vi "KE6514.constructor.vi"(0 "name":string, 2 "data in":string, 5 "error in (no error)":errorcluster) -> (14 "i ref out":refnum<vi>, 16 "data out":string, 19 "error out":errorcluster)   [LabVIEW 2014, in "KE6514.lvlib"]
doc: "This is the constructor of a class.\n\nLicense Agreement for this software:\n\nCopyright (C)\nGesellschaft für Schwerionenforschung, GSI\nPlanckstr. 1\n64291 Darmstadt\nGermany\n\nContact: D.Beck@gsi.de \n\nThis program is free software; you can redistribute it and/or modify it under the terms of the \nGNU General Public License as published by the Free Software Foundation; either version 2 of \nthe license, or (at your option) any later version.\n\nThis program is distributed in the hope that it will be useful, but WITHOUT ANY WARRANTY; \nwithout even the implied warranty of MERCHANTABILITY or FITNESS FOR A PARTICULAR PURPOSE. See the GNU General License for more details (http://www.gnu.org).\n\nGesellschaft für Schwerionenforschung, GSI\nPlanckstr. 1, 64291 Darmstadt, Germany\nFor all questions and ideas contact: M.Richter@gsi.de, H.Brand@gsi.de or D.Beck@gsi.de.\nLast update: 16-JUN-2004"
uses:
  KE6514.lvlib
  CSCore/CSApplicationBaseClasses/DeviceBase/DeviceBase.myEventNames.ctl
  CSCore/CSApplicationBaseClasses/DeviceBase/DeviceBase.lvlib
  CSCore/CSSystem/CSSystemLib/CSSystemLib.lvlib
  CSCore/BaseProcess/BaseProcess.lvlib
  CSlibraries-extern/DimLVEvent/LVDimInterface/LVDimInterface.lvlib
  CSinstr.lib/KE6514/KE6514Driver.lvlib
  CSCore/CSObj/CSObj.lvlib
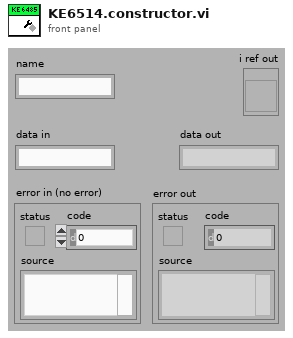
[diagram p1: front panel]
types:
  T1 = enum16{"SetAttribute", "GetAttribute", "CreateAttribute", "DestroyAttribute", "DestroyAllAtributes"}
  T2 = typedef "DeviceBase.lvlib/DeviceBase.myEventNames.ctl" = enum16{"lvmsg://Initialize", "lvmsg://Close", "lvmsg://Configure", "lvmsg://Reset", "lvmsg://IDQuery"}
  T3 = typedef "BaseProcess.lvlib/BaseProcess.i attribute.ctl" = cluster{"EventStatus":string, "EventError":i32, "PresetEvtWatchD":i32, "PresetPdcWatchD":i32, "EventTimeout":i32, "PeriodicInterval":i32, "Interface":string[], "Address":string[], "Special":string[], "PeriodicError":i32, "PeriodicStatus":string, "SuperProc":string, "Descriptors":T4[], "CaseRef":refnum<vi>, "PdcRef":refnum<vi>, "Thread Ref":refnum<vi>, "eventErrorID":i32, "eventStatusID":i32, "periodicErrorID":i32, "periodicStatusID":i32, "pdcCtrID":i32}
  T4 = typedef "BaseProcess.lvlib/BaseProcess.descriptor definition.ctl" = cluster{"selector":string, "descriptor":T5}
  T5 = typedef "BaseProcess.lvlib/BaseProcess.descriptor string definition.ctl" = string
  T6 = typedef "KE6514.lvlib/KE6514.i attribute.ctl" = cluster{"VISA resource name":refnum<visa-resource-name>, "ValueID":i32, "MeasurementRunning?":bool, "actSequencer":string, "actScanner":string, "actPPG":string, "MeasuredID":i32}
  T7 = cluster{"error":bool, "code":i32, "source":string}
  T8 = typedef "CSObj.lvlib/CSObj.i attribute.ctl" = cluster{"VI Refnum":refnum<vi>, "Front Panel Ref":refnum<vi>, "semaphore":T9, "date of birth":dbl, "ageID":i32, "systemID":i32, "classID":i32, "conditionID":i32, "DefaultPanelType":u16}
  T9 = typedef "Semaphore RefNum" = refnum<k1>
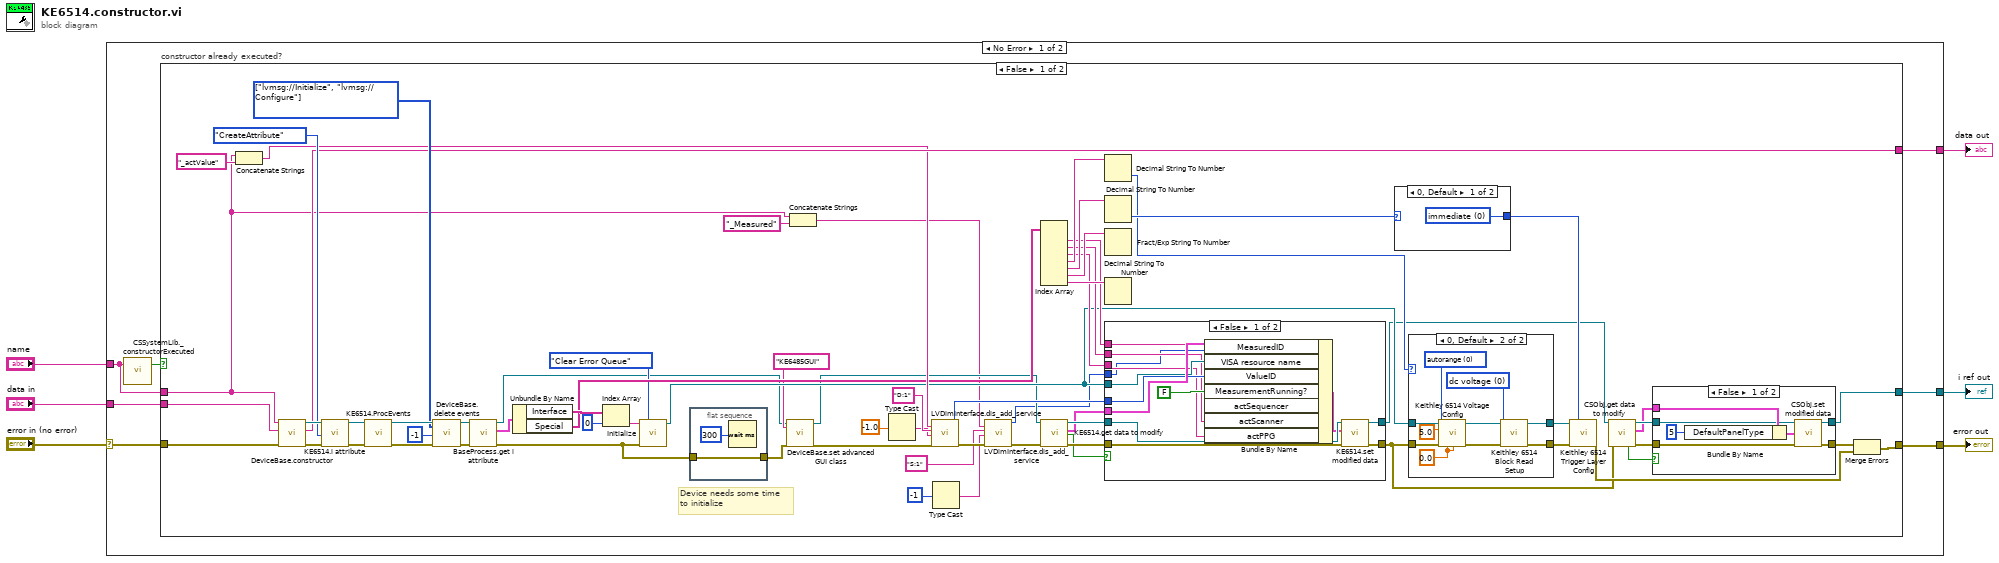
[diagram p0: block diagram]
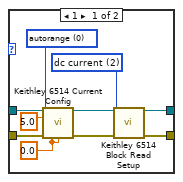
[diagram p3: hidden frame]
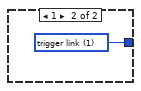
[diagram p4: hidden frame]
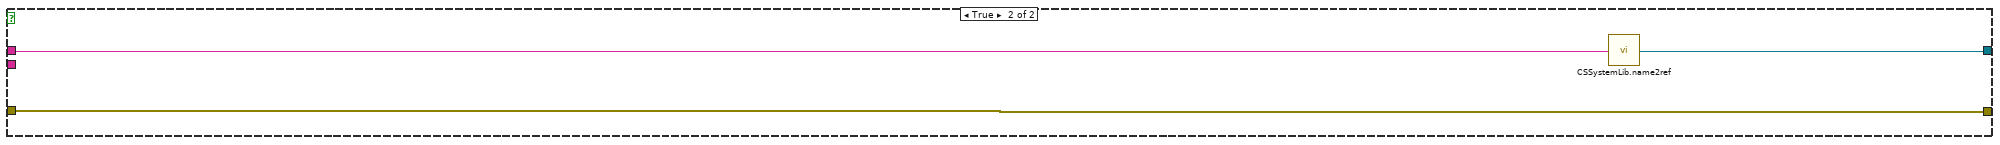
[diagram p6: hidden frame]
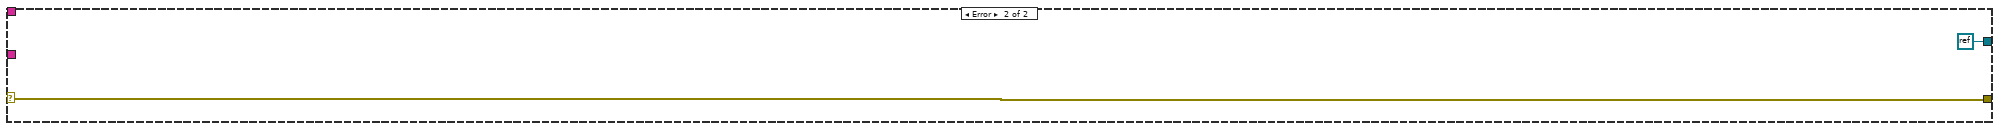
[diagram p7: hidden frame]
diagram:
  n1 = case shown="No Error" "error in (no error)" {
    selector: "error in (no error)" -> [w11 w133]
    tunnel: "name" -> [w10 _]
    tunnel: [w13 refnum<k0> refnum ("Not a Refnum Constant")] -> w5
    tunnel: [w12 w133] -> w4
    tunnel: "data in" -> [w8 _]
    tunnel: [w7 _] -> w1
    frame No Error {
      n2 = call "CSSystemLib._constructorExecuted.vi"("name"=w10) -> ("constructor executed?"=w9:bool)  [unwired: 18 in]
      n3 = case "constructor already executed?" shown="False" w9 {
        tunnel: w10 -> [w17 w132]
        tunnel: [w29 w131] -> w13
        tunnel: [w27 w130] -> w12
        tunnel: w11 -> [w76 w130]
        tunnel: w8 -> [w75 _]
        tunnel: [w70 _] -> w7
        frame False {
          w72 = T2[] [enum."lvmsg://Initialize", enum."lvmsg://Configure"] items=["lvmsg://Initialize", "lvmsg://Close", "lvmsg://Configure", "lvmsg://Reset", "lvmsg://IDQuery"] ("events")
          # "Device needs some time\nto initialize"
          n4 = Concatenate Strings(w17, "_actValue" ("string")) -> (w67:string)
          n5 = call "DeviceBase.constructor.vi"("name"=w17, "data in"=w75, "error in (no error)"=w76) -> ("i ref out"=w81:refnum<vi>, "data out"=w70:string, "error out"=w80:errorcluster)  [unwired: 14 in]
          n6 = call "KE6514.i attribute.vi"("VI Refnum"=w81, "Action"=T1."CreateAttribute", "error in (no error)"=w80) -> ("VI Refnum out"=w78:refnum<vi>, "error out"=w77:errorcluster)  [unwired: 14 in, 1 out]
          n7 = call "KE6514.ProcEvents.vi"("i ref in"=w78, "error in (no error)"=w77) -> ("i ref out"=w74:refnum<vi>, "error out"=w73:errorcluster)  [unwired: 16 in]
          n8 = call "DeviceBase.delete events.vi"("i ref in"=w74, "events"=w72, "ms timeout (10000)"=-1, "error in (no error)"=w73) -> ("i ref out"=w68:refnum<vi>, "error out"=w69:errorcluster)  [unwired: 13 in, 1 out]
          n9 = call "BaseProcess.get i attribute.vi"("i ref in"=w68, "error in (no error)"=w69) -> ("i ref out"=w36:refnum<vi>, "i attribute"=w65:T3, "error out"=w23:errorcluster)  [unwired: 15 in]
          n10 = Unbundle By Name(w65) -> ("Interface"=w64:string[], "Special"=w58:string[])
          n11 = Index Array(array=w64, index=0) -> (element=w46:string)
          n12 = call "Initialize.vi"("VISA resource name"=w46, "Error Queue Option"=enum16{"Clear Error Queue", "Error Query"}."Clear Error Queue", "error in (no error)"=w23) -> ("VISA resource name out"=w44:refnum<visa-resource-name>)  [unwired: 11 in, 1 out]
          n13 = flat-sequence {
            tunnel: [w83] -> w24
            tunnel: w23 -> [w83]
            frame #0 {
              n14 = Wait (ms)(milliseconds to wait=u32 300) -> ()  [unwired: 1 out]
            }
          }
          n15 = call "DeviceBase.set advanced GUI class.vi"("i ref in"=w36, "advancedGUIClass"="KE6485GUI", "error in (no error)"=w24) -> ("i ref out"=w35:refnum<vi>, "error out"=w38:errorcluster)  [unwired: 14 in, 1 out]
          n16 = Concatenate Strings(w17, "_Measured" ("string")) -> (w16:string)
          n17 = Type Cast(x=-1.0) -> (*(type *) &x=w56:string)  [unwired: 1 in]
          n18 = call "LVDimInterface.dis_add_service.vi"("serviceName"=w67, "typeDescriptor"="D:1", "data"=w56, "error in (no error)"=w38) -> ("my_serviceID"=w55:i32, "error out"=w20:errorcluster)  [unwired: 14 in]
          n19 = Type Cast(x=i16 -1) -> (*(type *) &x=w14:string)  [unwired: 1 in]
          n20 = call "LVDimInterface.dis_add_service.vi"("serviceName"=w16, "typeDescriptor"="S:1", "data"=w14, "error in (no error)"=w20) -> ("my_serviceID"=w19:i32, "error out"=w21:errorcluster)  [unwired: 14 in]
          n21 = Index Array(array=w58) -> (element #1=w49:string, element #2=w48:string, element #3=w47:string, element #4=w50:string, element #5=w51:string, element #6=w52:string, element #7=w53:string)  [unwired: 7 in]
          n22 = call "KE6514.get data to modify.vi"("i ref in"=w35, "error in (no error)"=w21) -> ("i ref out"=w62:refnum<vi>, "i attribute"=w59:T6, "timed out"=w60:bool, "error out"=w61:errorcluster)  [unwired: 14 in]
          n23 = Decimal String To Number(string=w50) -> (number=w39:i32)  [unwired: 2 in, 1 out]
          n24 = Decimal String To Number(string=w51) -> (number=w41:i32)  [unwired: 2 in, 1 out]
          n25 = Fract/Exp String To Number(string=w52) -> ()  [unwired: 3 in, 2 out]
          n26 = Decimal String To Number(string=w53) -> ()  [unwired: 2 in, 2 out]
          n27 = case shown="False" w60 {
            tunnel: w62 -> [w127 w129]
            tunnel: [w126 w129] -> w30
            tunnel: w61 -> [w125 w128]
            tunnel: [w124 w128] -> w25
            tunnel: w59 -> [w123 _]
            tunnel: w44 -> [w121 _]
            tunnel: w55 -> [w120 _]
            tunnel: w49 -> [w118 _]
            tunnel: w48 -> [w117 _]
            tunnel: w47 -> [w116 _]
            tunnel: w19 -> [w115 _]
            frame False {
              n28 = Bundle By Name(cluster=w123, "MeasuredID"=w115, "VISA resource name"=w121, "ValueID"=w120, "MeasurementRunning?"=FALSE, "actSequencer"=w118, "actScanner"=w117, "actPPG"=w116) -> (w122:T6)
              n29 = call "KE6514.set modified data.vi"("i ref in"=w127, "i attribute"=w122, "error in (no error)"=w125) -> ("i ref out"=w126:refnum<vi>, "error out"=w124:errorcluster)  [unwired: 15 in]
            }
            frame True {
            }
          }
          n30 = case shown="0, Default" w41 {
            tunnel: [w113 w114] -> w40
            frame 0, Default {
              w113 = u16 0 items=["immediate", "trigger link"] ("source (imm:0)")
            }
            frame 1 {
              w114 = u16 1 items=["immediate", "trigger link"] ("source (imm:0)")
            }
          }
          n31 = case shown="0, Default" w39 {
            tunnel: w25 -> [w102 w112]
            tunnel: w44 -> [w101 w111]
            tunnel: [w96 w106] -> w43
            tunnel: [w95 w105] -> w42
            frame 1 {
              w93 = u16 2 items=["dc voltage", "resistance", "dc current", "charge"] ("function (Vdc:1)")
              w98 = u16 0 items=["autorange", "set min range", "set max range", "set range value"] ("range (autorange:0)")
              w99 = 0.0 ("Autorange Upper Limit (A) (21e-3)")
              n32 = call "Keithley 6514 Current Config.vi"("Resource In"=w101, "NPLC value (1.0)"=5.0, "range (autorange:0)"=w98, "error in (no error)"=w102, "Autorange Upper Limit (A) (21e-3)"=w99, "Autorange Lower Limit (A) (21e-12)"=w99) -> ("Resource Out (dupl)"=w97:refnum<visa-resource-name>, "error out"=w94:T7)  [unwired: 8 in]
              n33 = call "Keithley 6514 Block Read Setup.vi"("Resource In"=w97, "function (Vdc:1)"=w93, "error in (no error)"=w94) -> ("Resource Out (dupl)"=w96:refnum<visa-resource-name>, "error out"=w95:T7)  [unwired: 11 in]
            }
            frame 0, Default {
              w103 = u16 0 items=["dc voltage", "resistance", "dc current", "charge"] ("function (Vdc:1)")
              w108 = u16 0 items=["autorange", "set min range", "set max range", "set range value"] ("range (autorange:0)")
              w109 = 0.0 ("Autorange Upper Limit (A) (21e-3)")
              n34 = call "Keithley 6514 Voltage Config.vi"("Resource In"=w111, "NPLC value (1.00)"=5.0 ("NPLC value (1.0)"), "range (autorange:0)"=w108, "error in (no error)"=w112, "Autorange Upper Limit (V) (210)"=w109, "Autorange Lower Limit (V) (2.1)"=w109) -> ("Resource Out (dupl)"=w107:refnum<visa-resource-name>, "error out"=w104:T7)  [unwired: 8 in]
              n35 = call "Keithley 6514 Block Read Setup.vi"("Resource In"=w107, "function (Vdc:1)"=w103, "error in (no error)"=w104) -> ("Resource Out (dupl)"=w106:refnum<visa-resource-name>, "error out"=w105:T7)  [unwired: 11 in]
            }
          }
          n36 = call "Keithley 6514 Trigger Layer Config.vi"("Resource In"=w43, "error in (no error)"=w42, "source (imm:0)"=w40) -> ("error out"=w26:T7)  [unwired: 11 in, 1 out]
          n37 = call "CSObj.get data to modify.vi"("i ref in"=w30, "error in (no error)"=w25) -> ("i ref out"=w33:refnum<vi>, "i attribute"=w31:T8, "timed out"=w34:bool, "error out"=w32:errorcluster)  [unwired: 14 in]
          n38 = case shown="False" w34 {
            tunnel: [w88 w92] -> w29
            tunnel: w33 -> [w89 w92]
            tunnel: [w86 w91] -> w28
            tunnel: w32 -> [w87 w91]
            tunnel: w31 -> [w90 _]
            frame False {
              n39 = Bundle By Name(cluster=w90, "DefaultPanelType"=u16 5) -> (w85:T8)
              n40 = call "CSObj.set modified data.vi"("i ref in"=w89, "i attribute"=w85, "error in (no error)"=w87) -> ("i ref out"=w88:refnum<vi>, "error out"=w86:errorcluster)  [unwired: 15 in]
            }
            frame True {
            }
          }
          n41 = Merge Errors(w28, w26) -> (w27:errorcluster)
        }
        frame True {
          n42 = call "CSSystemLib.name2ref.vi"("name"=w132) -> ("obj refnum"=w131:refnum<vi>)
        }
      }
    }
    frame Error {
    }
  }
  "i ref out" <- w5
  "error out" <- w4
  "data out" <- w1
